vi "LoadModel.vi"(8 "error in (no error)":errorcluster, 10 "Actor In":refnum<class "Actor.lvclass">, 11 "GRMActor in":refnum<class "QPDController.lvclass">) -> (0 "error out":errorcluster, 3 "GRMActor out":refnum<class "QPDController.lvclass">)   [LabVIEW 2020, in "QPDController.lvlib" / "QPDController.lvclass"]
uses:
  QPDController.lvclass
  <vilib>/ActorFramework/Actor/Actor.lvclass
  Model/Hardware Layer/Simulation Hardware/DemoDAQ/DemoDAQ/DemoDAQ.lvclass
  E:/Development/DevHardSoftware/MicroscopyFramework/Model/Hardware Abstraction Layer/Component/DAQ/DAQ/DAQ.lvclass
  Model/Hardware Layer/Real Hardware/DAQ_QPT_Throlab/DAQ_QPT_Throlab/DAQ_QPD_Throlab.lvclass
  Model/Hardware Abstraction Layer/Component/DAQ/DAQ/DAQ.lvclass
  C:/Program Files/National Instruments/LabVIEW 2020/vi.lib/ActorFramework/Actor/Actor.lvclass
  Model/Hardware Abstraction Layer/Component/GenericActor/GenericActor/GenericController.lvclass
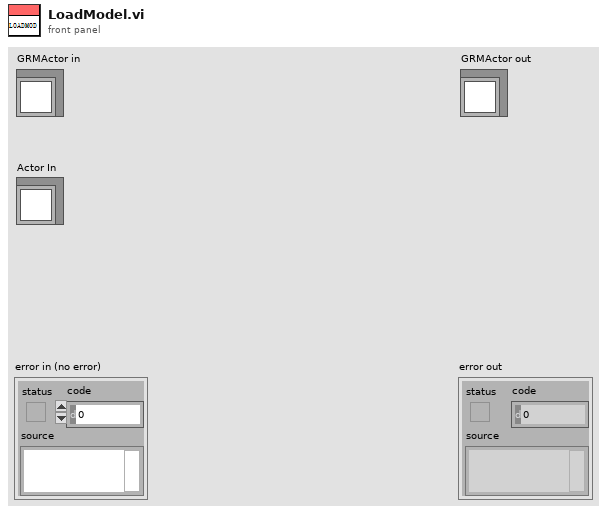
[diagram p1: front panel]
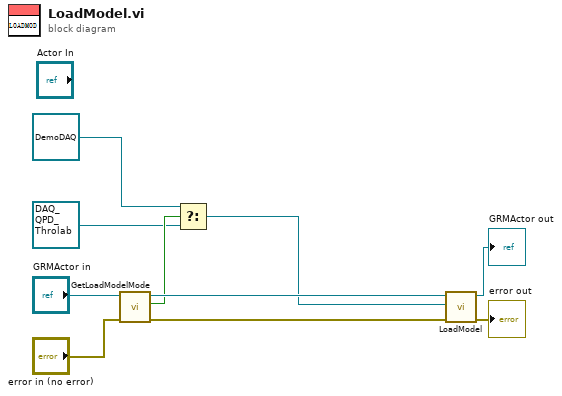
[diagram p0: block diagram]
diagram:
  n1 = call-dynamic "GetLoadModelMode.vi"("error in (no error)"="error in (no error)", "GenericController in"="GRMActor in") -> ("error out"=w7:errorcluster, "LoadDemoModel"=w4:bool, "GenericController out"=w5:refnum<class "QPDController.lvclass">)  [unwired: 7 in]
  n2 = Select(t=refnum<class "DemoDAQ.lvclass"> refnum ("DemoDAQ.lvlib:DemoDAQ.lvclass"), s=w4, f=refnum<class "DAQ_QPD_Throlab.lvclass"> refnum ("DAQ_QPD_Throlab.lvlib:DAQ_QPD_Throlab.lvclass")) -> (s? t:f=w2:refnum<class "DAQ.lvclass">)
  n3 = call-parent "LoadModel.vi"("error in (no error)"=w7, "Actor In"=w2, "GRMActor in"=w5) -> ("error out"=→"error out":errorcluster, "GRMActor out"=→"GRMActor out":refnum<class "QPDController.lvclass">)  [unwired: 7 in]
